vi "Emergency Abort.vi"(8 "Error In":errorcluster) -> (0 "Error Out":errorcluster)   [LabVIEW 2024]
doc: "This VI aborts all VIs that are running in the Application Instance.\n\nRecommended use: Run this VI when your application becomes irresponsive, or when you want to \"kill\" all VIs that may be running silently in the background."
panel:
  out "Callers' Names":string[][](array[string])
  out "Loop iteration":i32
  out "VIs that were aborted directly (part 2)":string[](array[string])
  out "VIs that were aborted directly (part 1)":string[](array[string])
  # "Input\nInputs to the VI"
  # "Development\nControls or indicators that are useful for development or testing, but which are not outputs of the VI."
  # "Output\nOutputs of the VI"
  # "Emergency Abort"
  # "subVIs of the \"directly aborted\" VIs may have also been aborted."
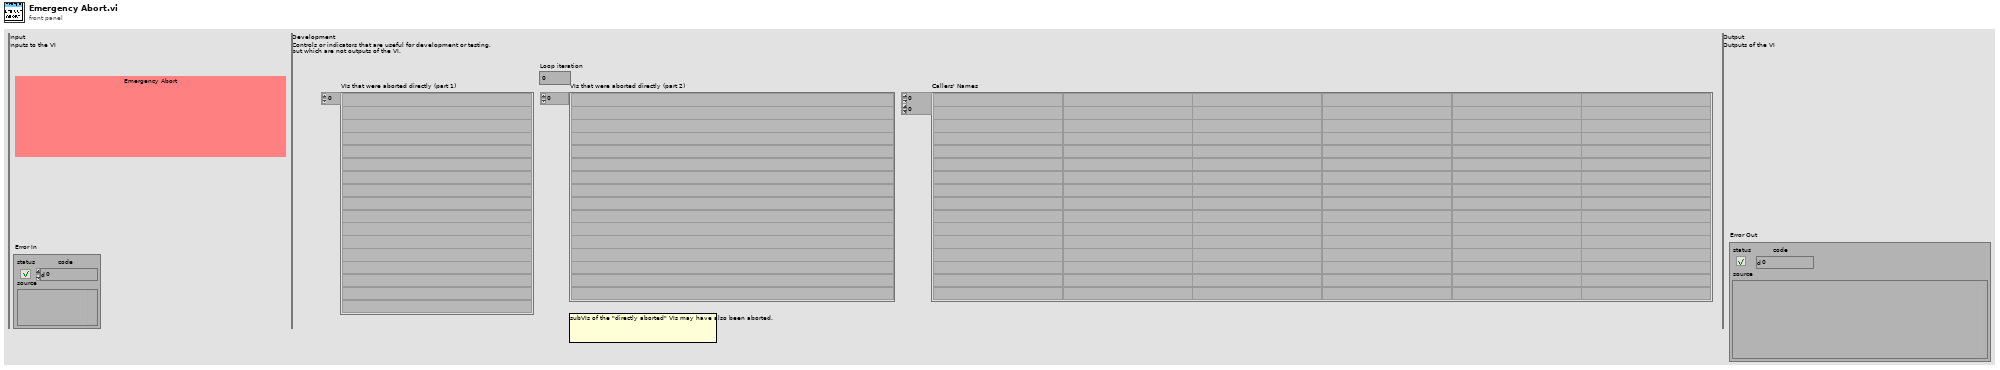
[diagram p1: front panel]
types:
  T1 = enum32{"Bad", "Idle", "Run top level", "Running"}
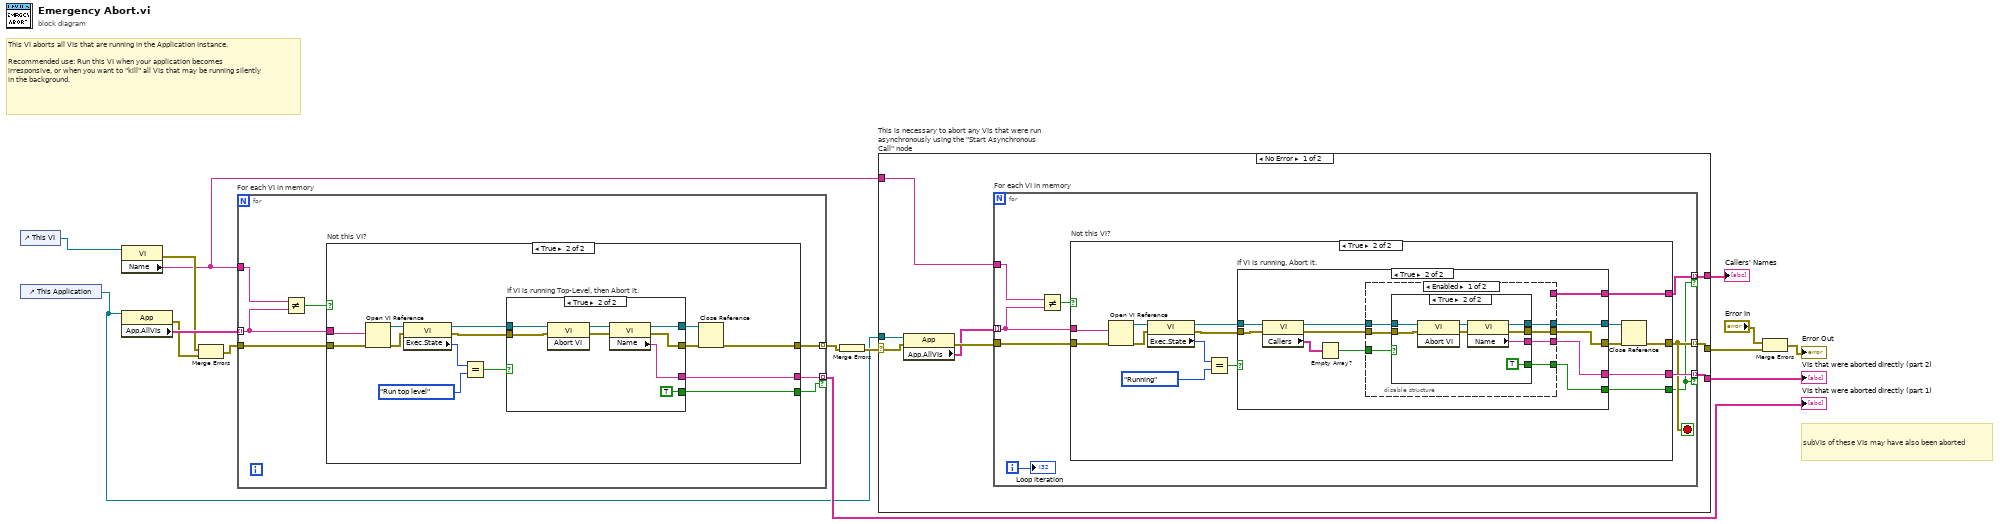
[diagram p0: block diagram]
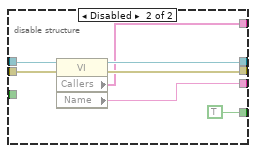
[diagram p5: hidden frame]
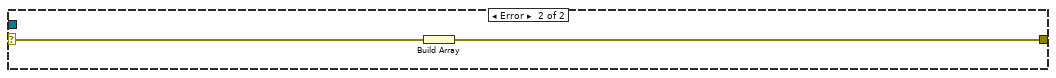
[diagram p6: hidden frame]
diagram:
  # "subVIs of these VIs may have also been aborted"
  # "This VI aborts all VIs that are running in the Application Instance.\n\nRecommended use: Run this VI when your application becomes irresponsive, or when you want to \"kill\" all VIs that may be running silently in the background."
  n1 = control-ref of="This VI"() -> (w14:refnum<vi>)
  n2 = control-ref of="This Application"() -> (w4:refnum<vi>)
  n3 = property class="VI"(reference=w14) -> (error out=w8:errorcluster, "Name"=w3:string)  [unwired: 1 in, 1 out]
  n4 = property class="App"(reference=w4) -> (error out=w7:errorcluster, "App.AllVIs"=w13:string[])  [unwired: 1 in, 1 out]
  n5 = Merge Errors(w8, w7) -> (w6:errorcluster)
  n6 = for "For each VI in memory" {
    tunnel: w3 -> [w22]
    tunnel: w13 -> [w20] mode=indexing
    tunnel: [w19] -> w12 mode=indexing
    tunnel: [w18] -> w9 mode=indexing if=w17
    tunnel: w6 -> [w16]
    n7 = Not Equal?(x=w22, y=w20) -> (x != y?=w21:bool)
    n8 = case "Not this VI?" shown="True" w21 {
      tunnel: w20 -> [_ w37]
      tunnel: [w23 w27] -> w19
      tunnel: [_ w26] -> w18
      tunnel: [_ w25] -> w17
      tunnel: w16 -> [w23 w24]
      frame False {
      }
      frame True {
        n9 = Open VI Reference(vi path=w37, error in (no error)=w24) -> (vi reference=w36:refnum<vi>, error out=w28:errorcluster)  [unwired: 4 in]
        n10 = property class="VI"(reference=w36, error in=w28) -> (reference out=w32:refnum<vi>, error out=w29:errorcluster, "Exec.State"=w35:T1)
        n11 = Equal?(x=w35, y=T1."Run top level") -> (x = y?=w33:bool)
        n12 = case "If VI is running Top-Level, then Abort it." shown="True" w33 {
          tunnel: w32 -> [w38 w47]
          tunnel: [w38 w42] -> w31
          tunnel: [w39 w44] -> w30
          tunnel: w29 -> [w39 w45]
          tunnel: [_ w41] -> w26
          tunnel: [_ TRUE] -> w25
          frame False {
          }
          frame True {
            n13 = invoke class="VI" method="Abort VI"(reference=w47, error in=w45) -> (reference out=w43:refnum<vi>, error out=w46:errorcluster)  [unwired: 1 in, 1 out]
            n14 = property class="VI"(reference=w43, error in=w46) -> (reference out=w42:refnum<vi>, error out=w44:errorcluster, "Name"=w41:string)
          }
        }
        n15 = Close Reference(reference=w31, error in (no error)=w30) -> (error out=w27:errorcluster)
      }
    }
  }
  "VIs that were aborted directly (part 1)" <- w9
  n16 = Merge Errors(w12) -> (w10:errorcluster)
  n17 = case "This is necessary to abort any VIs that were run asynchronously using the \"Start Asynchronous Call\" node" shown="No Error" w10 {
    selector: w10 -> [w54 w119]
    tunnel: [w55 w118] -> w5
    tunnel: w4 -> [w52 _]
    tunnel: w3 -> [w51 _]
    tunnel: [w49 _] -> w1
    tunnel: [w48 _] -> w2
    frame No Error {
      n18 = property class="App"(reference=w52, error in=w54) -> (error out=w53:errorcluster, "App.AllVIs"=w50:string[])  [unwired: 1 out]
      n19 = for "For each VI in memory" {
        tunnel: w51 -> [w64]
        tunnel: w50 -> [w62] mode=indexing
        tunnel: [w58] -> w55 mode=indexing
        tunnel: [w61] -> w49 mode=indexing if=w56
        tunnel: w53 -> [w60]
        tunnel: [w57] -> w48 mode=indexing if=w56
        i -> [w59]
        stop <- w58 stop-if-true
        n20 = Not Equal?(x=w64, y=w62) -> (x != y?=w63:bool)
        n21 = case "Not this VI?" shown="True" w63 {
          tunnel: w62 -> [_ w80]
          tunnel: [w65 w73] -> w58
          tunnel: [_ w72] -> w61
          tunnel: [_ w71] -> w56
          tunnel: w60 -> [w65 w70]
          tunnel: [_ w66] -> w57
          frame False {
          }
          frame True {
            n22 = Open VI Reference(vi path=w80, error in (no error)=w70) -> (vi reference=w79:refnum<vi>, error out=w74:errorcluster)  [unwired: 4 in]
            n23 = property class="VI"(reference=w79, error in=w74) -> (reference out=w78:refnum<vi>, error out=w75:errorcluster, "Exec.State"=w68:T1)
            n24 = Equal?(x=w68, y=T1."Running") -> (x = y?=w69:bool)
            n25 = case "If VI is running, Abort it." shown="True" w69 {
              tunnel: w78 -> [w81 w87]
              tunnel: [w81 w92] -> w77
              tunnel: [w82 w93] -> w76
              tunnel: w75 -> [w82 w89]
              tunnel: [_ w91] -> w72
              tunnel: [_ w83] -> w71
              tunnel: [_ w90] -> w66
              frame False {
              }
              frame True {
                n26 = property class="VI"(reference=w87, error in=w89) -> (reference out=w86:refnum<vi>, error out=w88:errorcluster, "Callers"=w85:string[])
                n27 = Empty Array?(array=w85) -> (empty?=w84:bool)
                n28 = disable-structure shown="Enabled" {
                  disable-tunnel: w86 -> [w100 w115]
                  disable-tunnel: w88 -> [w99 w117]
                  disable-tunnel: [w98 w116] -> w93
                  disable-tunnel: [w97 w114] -> w92
                  disable-tunnel: [w96 w112] -> w91
                  disable-tunnel: [_ w113] -> w90
                  disable-tunnel: w84 -> [w95 _]
                  disable-tunnel: [w94 TRUE] -> w83
                  frame Enabled {
                    n29 = case shown="True" w95 {
                      tunnel: w100 -> [w101 w110]
                      tunnel: w99 -> [w102 w108]
                      tunnel: [w102 w107] -> w98
                      tunnel: [w101 w105] -> w97
                      tunnel: [_ w104] -> w96
                      tunnel: [_ TRUE] -> w94
                      frame False {
                      }
                      frame True {
                        n30 = invoke class="VI" method="Abort VI"(reference=w110, error in=w108) -> (reference out=w106:refnum<vi>, error out=w109:errorcluster)  [unwired: 1 in, 1 out]
                        n31 = property class="VI"(reference=w106, error in=w109) -> (reference out=w105:refnum<vi>, error out=w107:errorcluster, "Name"=w104:string)
                      }
                    }
                  }
                  frame Disabled {
                    n32 = property class="VI"(reference=w115, error in=w117) -> (reference out=w114:refnum<vi>, error out=w116:errorcluster, "Callers"=w113:string[], "Name"=w112:string)
                  }
                }
              }
            }
            n33 = Close Reference(reference=w77, error in (no error)=w76) -> (error out=w73:errorcluster)
          }
        }
        "Loop iteration" <- w59
      }
    }
    frame Error {
      n34 = Build Array(w119) -> (w118:errorcluster[])
    }
  }
  "VIs that were aborted directly (part 2)" <- w1
  "Callers' Names" <- w2
  n35 = Merge Errors("Error In", w5) -> (→"Error Out":errorcluster)
